vi "GetNamedUnbundlerReference.vi"(8 "error in":errorcluster, 11 "NamedBundler in":refnum<class "NamedUnbundler.lvclass">) -> (0 "error out":errorcluster, 1 "reference out":refnum<vi>, 3 "NamedBundler out":refnum<class "NamedUnbundler.lvclass">)   [LabVIEW 2014, in "NamedUnbundler.lvclass"]
uses:
  NamedUnbundler.lvclass
  Generic/Generic.lvclass
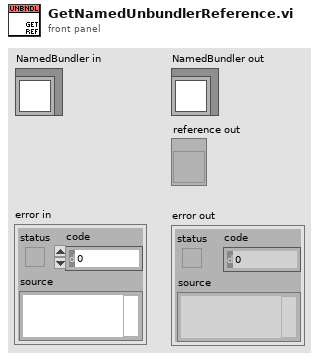
[diagram p1: front panel]
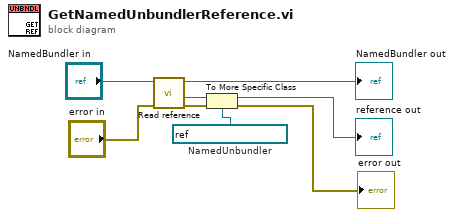
[diagram p0: block diagram]
diagram:
  w8 = refnum<vi> refnum  # NamedUnbundler
  n1 = call "Read reference.vi"("error in"="error in", "GObject in"="NamedBundler in") -> ("error out"=w7:errorcluster, "reference"=w6:refnum<vi>, "GObject out"=→"NamedBundler out":refnum<class "NamedUnbundler.lvclass">)  [unwired: 5 in]
  n2 = To More Specific Class(target class=w8, reference=w6, error in=w7) -> (specific class reference=→"reference out":refnum<vi>, error out=→"error out":errorcluster)
